vi "DriveGetGyroZero.vi"() -> (3 "GyroZero":dbl)   [LabVIEW 2020]
doc: "Get GyroZero from drive for use elsewhere\n\nOutputs:\n-- GyroZero -- Double -- gets gyro zero from drive global"
uses:
  DriveGlobal.vi
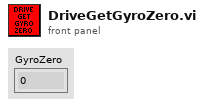
[diagram p1: front panel]
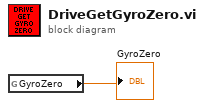
[diagram p0: block diagram]
diagram:
  n1 = global read "DriveGlobal.vi" "GyroZero"() -> (→"GyroZero":dbl)
